vi "S4ACS_Controller.vi"() -> ()   [LabVIEW 2018]
uses:
  Channel Manager/Channel Manager.lvclass
  Channel/Channel.lvclass
panel:
  in  "Stop Button":bool
  in  "Camera ID":u8=1
  in  "Channel Manager.lvclass":refnum<class "Channel Manager.lvclass">
  out "GUI Message":string
  out "Error":string
  # "Welcome to the\nAcquisition Control System (ACS)\nof the SPARC4 instrument"
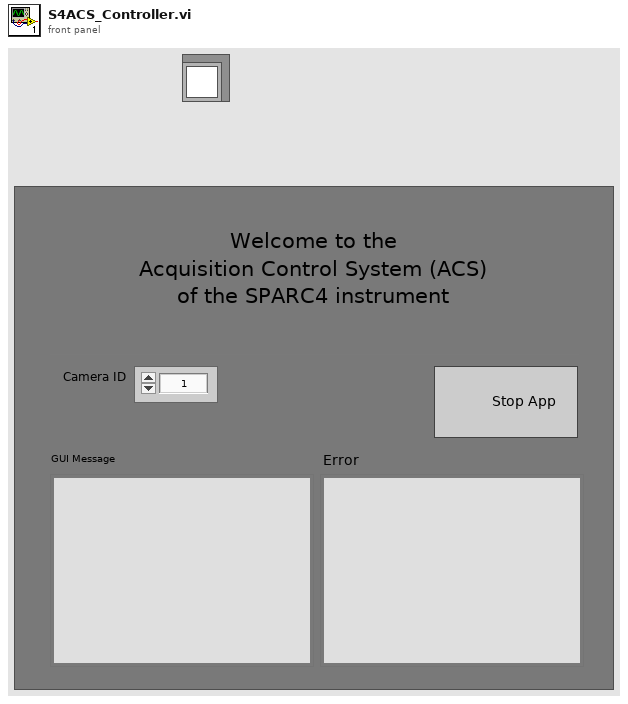
[diagram p1: front panel]
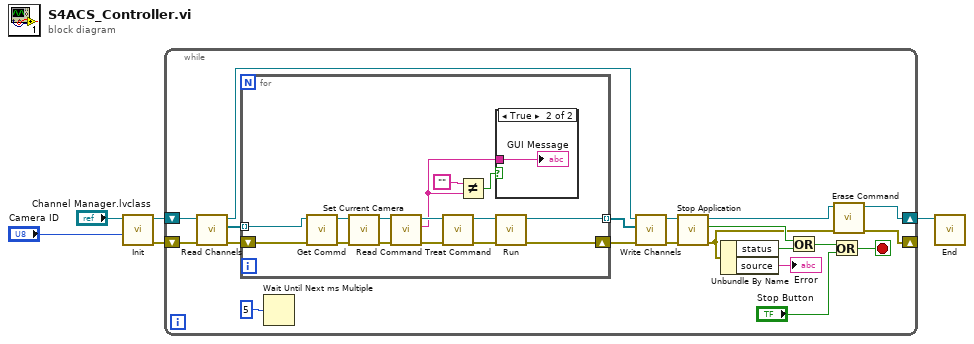
[diagram p0: block diagram]
diagram:
  n1 = call "Init.vi"("Computer Specifier"="Camera ID", "Channel Manager in"="Channel Manager.lvclass") -> ("error out"=w4:errorcluster, "Channel Manager out"=w5:refnum<class "Channel Manager.lvclass">)  [unwired: 8 in]
  n2 = while {
    shift-right: [w8] -> _
    shift-left: w4 -> [w11]
    shift-right: [w9] -> w3
    shift-left: w5 -> [w12]
    stop <- w13 stop-if-true
    n3 = call "Read Channels.vi"("error in (no error)"=w11, "Channel Manager in"=w12) -> ("error out"=w24:errorcluster, "Array"=w25:refnum<class "Channel.lvclass">[], "Channel Manager out"=w22:refnum<class "Channel Manager.lvclass">)  [unwired: 7 in]
    n4 = for {
      tunnel: w25 -> [w37] mode=indexing
      tunnel: [w30] -> w23 mode=indexing
      shift-right: [w29] -> w21
      shift-left: w24 -> [w38]
      n5 = call "Get Commd.vi"("error in (no error)"=w38, "Channel in"=w37) -> ("error out"=w31:errorcluster, "Channel out"=w32:refnum<class "Channel.lvclass">)  [unwired: 8 in]
      n6 = call "Set Current Camera.vi"("error in (no error)"=w31, "Channel in"=w32) -> ("error out"=w40:errorcluster, "Channel out"=w39:refnum<class "Channel.lvclass">)  [unwired: 8 in]
      n7 = call "Read Command.vi"("error in (no error)"=w40, "Channel in"=w39) -> ("error out"=w34:errorcluster, "Message"=w27:string, "Channel out"=w35:refnum<class "Channel.lvclass">)  [unwired: 7 in]
      n8 = call "Treat Command.vi"("error in (no error)"=w34, "Channel in"=w35) -> ("error out"=w33:errorcluster, "Channel out"=w36:refnum<class "Channel.lvclass">)  [unwired: 8 in]
      n9 = Not Equal?(x="", y=w27) -> (x != y?=w28:bool)
      n10 = case shown="True" w28 {
        tunnel: w27 -> [_ w41]
        frame False {
        }
        frame True {
          "GUI Message" <- w41
        }
      }
      n11 = call "Run.vi"("error in (no error)"=w33, "Channel in"=w36) -> ("error out"=w29:errorcluster, "Channel out"=w30:refnum<class "Channel.lvclass">)  [unwired: 8 in]
    }
    n12 = Wait Until Next ms Multiple(millisecond multiple=u32 5) -> ()  [unwired: 1 out]
    n13 = call "Write Channels.vi"("error in (no error)"=w21, "Channels Array"=w23, "Channel Manager in"=w22) -> ("error out"=w20:errorcluster, "Channel Manager out"=w19:refnum<class "Channel Manager.lvclass">)  [unwired: 7 in]
    n14 = call "Stop Application.vi"("error in (no error)"=w20, "Channel Manager in"=w19) -> ("error out"=w7:errorcluster, "Stop Application"=w17:bool, "Channel Manager out"=w6:refnum<class "Channel Manager.lvclass">)  [unwired: 7 in]
    n15 = Unbundle By Name(w7) -> ("status"=w18:bool, "source"=→"Error":string)
    n16 = Or(x=w17, y=w18) -> (x .or. y?=w15:bool)
    n17 = Or(x=w15, y="Stop Button") -> (x .or. y?=w13:bool)
    n18 = call "Erase Command.vi"("error in (no error)"=w7, "Channel Manager in"=w6) -> ("error out"=w8:errorcluster, "Channel Manager out"=w9:refnum<class "Channel Manager.lvclass">)  [unwired: 8 in]
  }
  n19 = call "End.vi"("Channel Manager in"=w3) -> ()  [unwired: 9 in, 2 out]
